vi "SetBottomSize.vi"(8 "error in (no error)":errorcluster, 10 "Bottom Pane Size":i32, 11 "PentaPanesGUI in":refnum<class "PentaPanes.lvclass">) -> (0 "error out":errorcluster, 3 "PentaPanesGUI out":refnum<class "PentaPanes.lvclass">)   [LabVIEW 2022 SP3, in "PentaPanesLibrary.lvlib" / "PentaPanes.lvclass"]
doc: "This VI sets the height of the bottom pane.\n\nBottom Pane Size - The height of the pane to be set."
uses:
  PentaPanes.lvclass
  PentaPanes.lvclass/PentaPanes.ctl
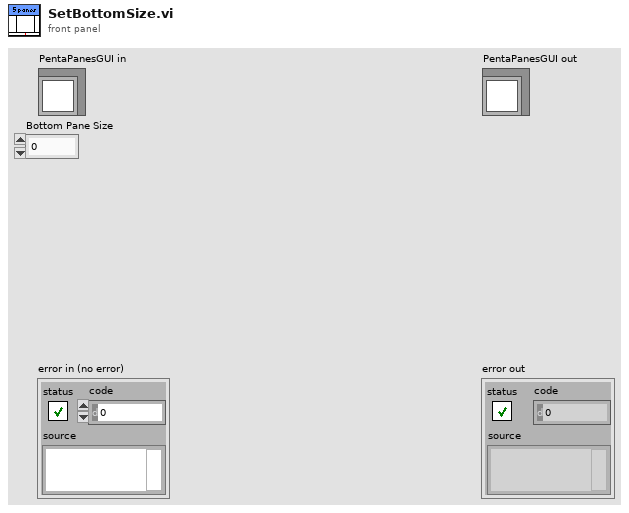
[diagram p1: front panel]
types:
  T1 = typedef "PentaPanesLibrary.lvlib/PentaPanes.lvclass/SplittersCluster.ctl" = cluster{"Top Splitter":refnum<vi>, "Left Splitter":refnum<vi>, "Right Splitter":refnum<vi>, "Bottom Splitter":refnum<vi>}
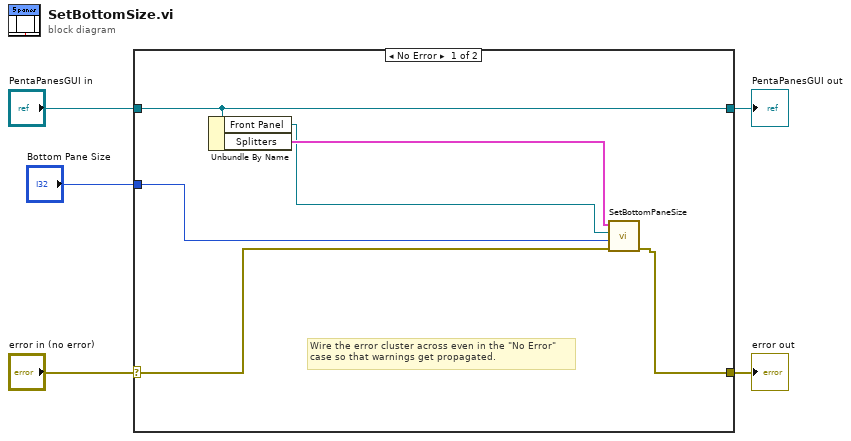
[diagram p0: block diagram]
diagram:
  n1 = case shown="No Error" "error in (no error)" {
    selector: "error in (no error)" -> [w7 w13]
    tunnel: [w6 w13] -> w4
    tunnel: [w11 w12] -> w2
    tunnel: "PentaPanesGUI in" -> [w11 w12]
    tunnel: "Bottom Pane Size" -> [w8 _]
    frame No Error {
      # "Wire the error cluster across even in the \"No Error\"\ncase so that warnings get propagated."
      n2 = Unbundle By Name(w11) -> ("Front Panel"=w9:refnum<vi>, "Splitters"=w10:T1)
      n3 = call "SetBottomPaneSize.vi"("error in (no error)"=w7, "Bottom Pane Size"=w8, "Front Panel"=w9, "Splitters"=w10) -> ("error out"=w6:errorcluster)  [unwired: 7 in]
    }
    frame Error {
    }
  }
  "error out" <- w4
  "PentaPanesGUI out" <- w2
